vi "Test Get Count and Get End Offset.vi"() -> ()   [LabVIEW 2021]
uses:
  pcap_Parse_Build_CIF.lvclass/pcap_Parse_Build_CIF.ctl
  Build/SubVIs/Flatten Packet Header.vi
  <vilib>/CIF Foundation/CIF Utilities/DataTypes/Flatten Unflatten/Unflatten U32.vi
  <vilib>/CIF Foundation/CIF Utilities/DataTypes/Flatten Unflatten/Flatten U32.vi
  pcap_Parse_Build_CIF.lvclass
panel:
  out "pass":bool
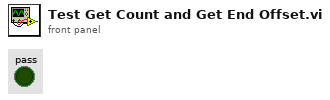
[diagram p1: front panel]
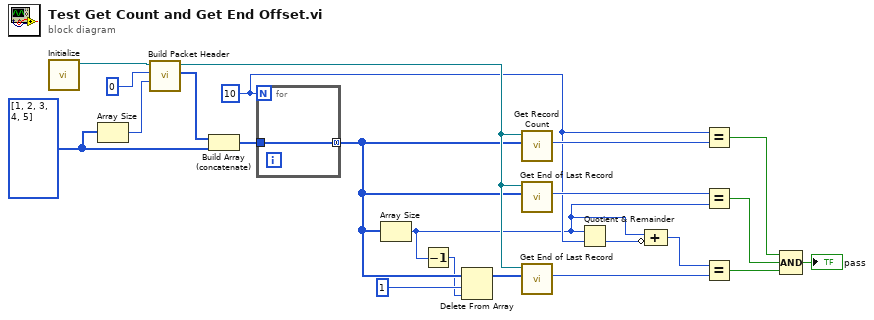
[diagram p0: block diagram]
diagram:
  w9 = 10
  w16 = u8[] [1, 2, 3, 4, 5] ("element")
  n1 = call "Initialize.vi"() -> ("pcap Parse and Build out"=w20:refnum<class "pcap_Parse_Build_CIF.lvclass">)  [unwired: 11 in]
  n2 = Array Size(array=w16) -> (size(s)=w15:i32)
  n3 = call "Build Packet Header.vi"("Length"=w15, "TAI Time (ns)"=i64 0, "pcap Parse and Build in"=w20) -> ("Flattened Data out"=w22:u8[], "pcap Parse and Build out"=w13:refnum<class "pcap_Parse_Build_CIF.lvclass">)  [unwired: 7 in]
  n4 = Build Array (concatenate)(w22, w16) -> (w19:u8[])
  n5 = for {
    N: w9 -> [_]
    tunnel: w19 -> [w23]
    tunnel: [w23] -> w12 mode=concatenating
  }
  n6 = Array Size(array=w12) -> (size(s)=w8:i32)
  n7 = Decrement(x=w8) -> (x-1=w10:i32)
  n8 = Delete From Array(array=w12, length=1, index=w10) -> (array with subset deleted=w17:u8[])  [unwired: 1 out]
  n9 = call "Get Record Count.vi"("Bytes in"=w12, "pcap_Parse_Build_CIF"=w13) -> ("Records"=w14:i32)  [unwired: 9 in]
  n10 = call "Get End of Last Record.vi"("Bytes in"=w12, "pcap_Parse_Build_CIF"=w13) -> ("End Offset"=w11:i32)  [unwired: 9 in]
  n11 = call "Get End of Last Record.vi"("Bytes in"=w17, "pcap_Parse_Build_CIF"=w13) -> ("End Offset"=w6:i32)  [unwired: 9 in]
  n12 = Quotient & Remainder(x=w8, y=w9) -> (floor(x/y)=w7:i32)  [unwired: 1 out]
  n13 = Compound Arithmetic op=ADD(w8, invert w7) -> (w5:i32)
  n14 = Equal?(x=w9, y=w14) -> (x = y?=w2:bool)
  n15 = Equal?(x=w11, y=w8) -> (x = y?=w3:bool)
  n16 = Equal?(x=w5, y=w6) -> (x = y?=w4:bool)
  n17 = Compound Arithmetic op=AND(w2, w3, w4) -> (→"pass":bool)
